vi "Read Test Configuration (INI) File.vi"() -> (1 "Filename":string, 2 "Filepath":path, 3 "Experiments":T1={"Exp 1"={"P2_Sweep_Stop_V"=36.0, "P2_Sweep_Step_V"=1.0, "Experiment Name"="", "Resistance Threshold"=1.0, "P1_Fixed_Voltage"=36.0, "P2_Sweep_Start_V"=36.0}, "Exp 3"={"P2_Sweep_Stop_V"=36.0, "P2_Sweep_Step_V"=1.0, "Experiment Name"="", "Resistance Threshold"=1.0, "P1_Fixed_Voltage"=36.0, "P2_Sweep_Start_V"=36.0}, "Exp 2"={"P2_Sweep_Stop_V"=36.0, "P2_Sweep_Step_V"=1.0, "Experiment Name"="", "Resistance Threshold"=1.0, "P1_Fixed_Voltage"=36.0, "P2_Sweep_Start_V"=36.0}, "Exp 4"={"P2_Sweep_Stop_V"=36.0, "P2_Sweep_Step_V"=1.0, "Experiment Name"="", "Resistance Threshold"=1.0, "P1_Fixed_Voltage"=36.0, "P2_Sweep_Start_V"=36.0}})   [LabVIEW 2013]
doc: "Read Test Configuration file. Set Cluster Output which SDR will choose from later."
uses:
  Support/Controls/Multiple Exp Setup.ctl
  Support/Controls/Individual User Inputs.ctl
  <vilib>/Utility/config.llb/Read Key (Double).vi
  <vilib>/Utility/config.llb/Read Key (String).vi
  <vilib>/Utility/config.llb/Read Key (Path).vi
  <vilib>/Utility/config.llb/NI_LVConfig.lvlib
panel:
  # "Test Settings"
  # "Make the Stop and Step Negative \nfor negative sweep"
  # "Calculation Settings"
  # "Test Settings"
  # "Make the Stop and Step Negative \nfor negative sweep"
  # "Calculation Settings"
  # "Test Settings"
  # "Make the Stop and Step Negative \nfor negative sweep"
  # "Calculation Settings"
  # "Test Settings"
  # "Make the Stop and Step Negative \nfor negative sweep"
  # "Calculation Settings"
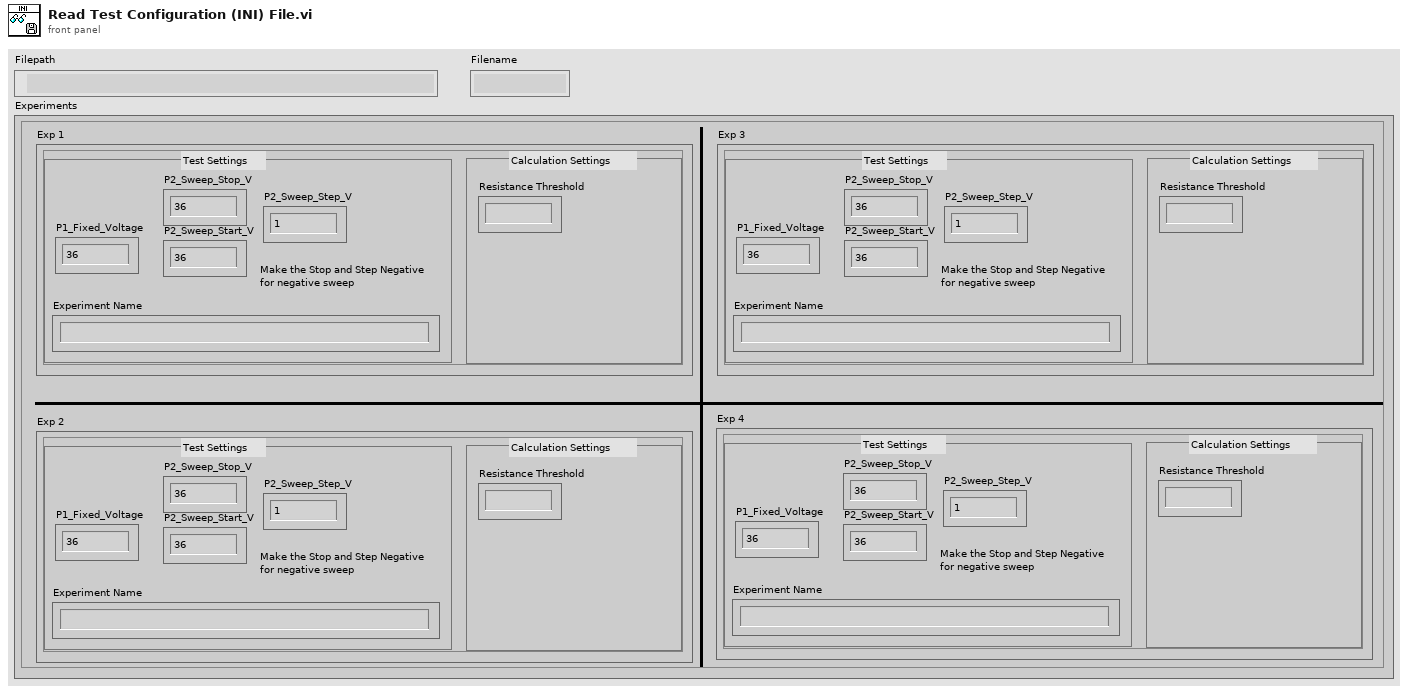
[diagram p1: front panel]
types:
  T1 = typedef "Multiple Exp Setup.ctl" = cluster{"Exp 1":T2, "Exp 3":T2, "Exp 2":T2, "Exp 4":T2}
  T2 = typedef "Individual User Inputs.ctl" = cluster{"P2_Sweep_Stop_V":dbl, "P2_Sweep_Step_V":dbl, "Experiment Name":string, "Resistance Threshold":dbl, "P1_Fixed_Voltage":dbl, "P2_Sweep_Start_V":dbl}
  T3 = typedef "NI_LVConfig.lvlib/Config Data RefNum.ctl" = refnum<k1>
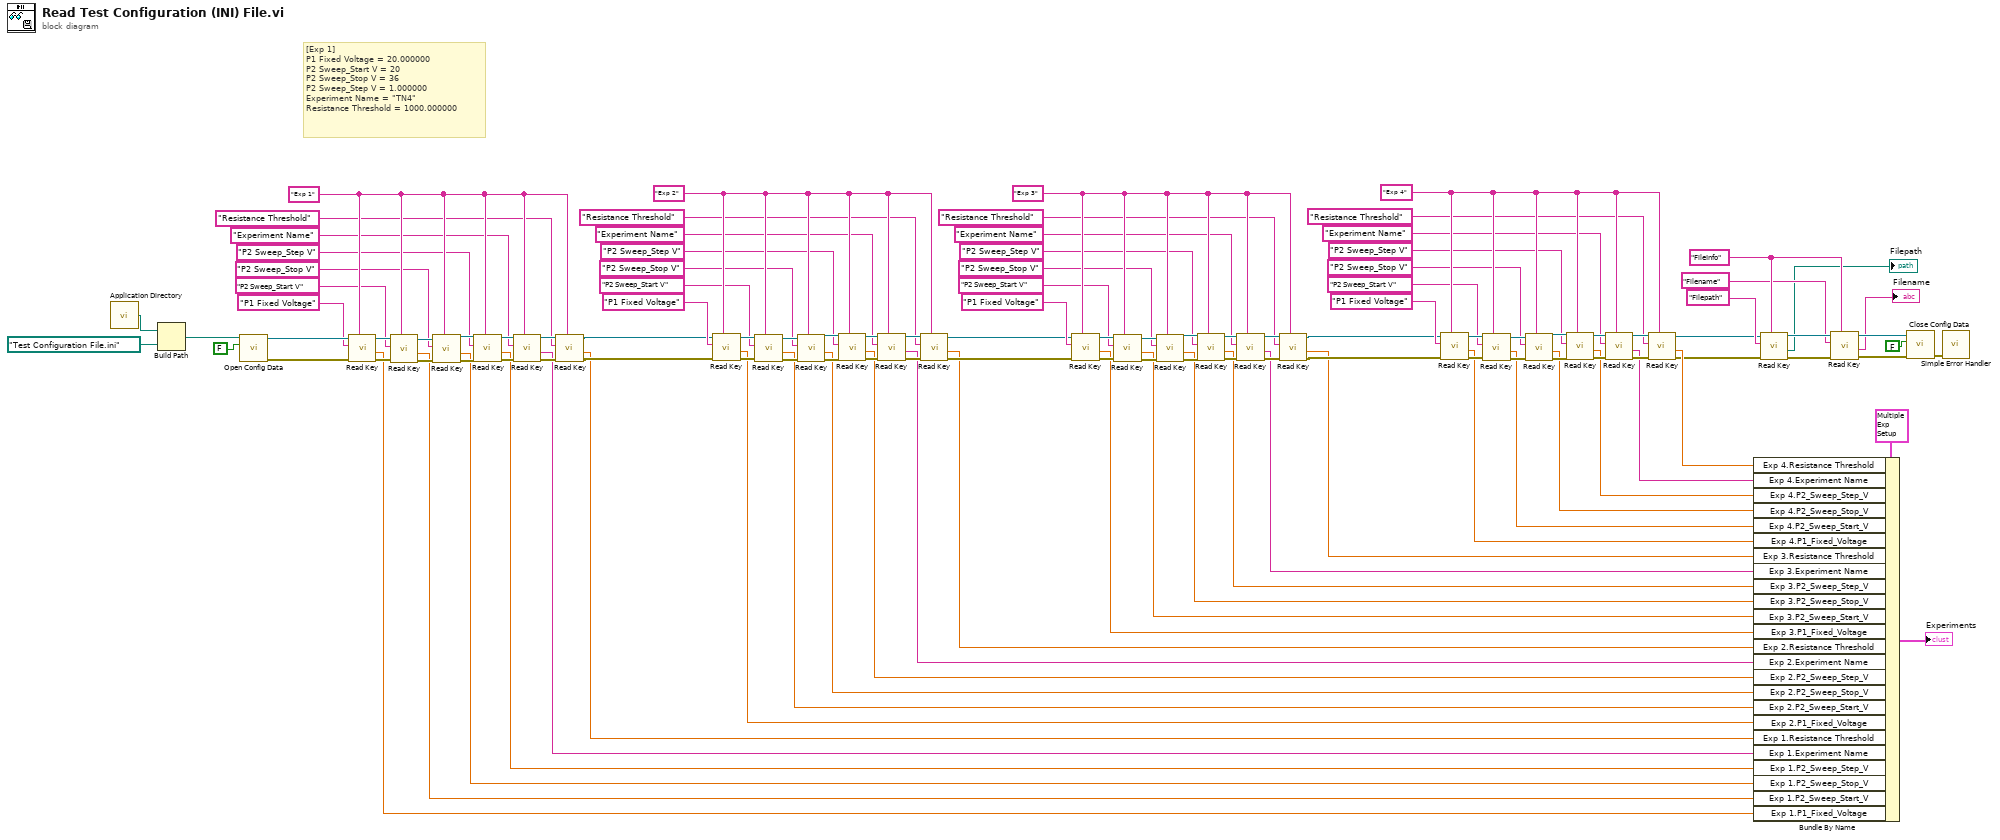
[diagram p0: block diagram]
diagram:
  w8 = "FileInfo" ("section")
  w44 = "Exp 4" ("section")
  w63 = "Exp 3" ("section")
  w82 = "Exp 2" ("section")
  w99 = "Exp 1" ("section")
  # "[Exp 1]\nP1 Fixed Voltage = 20.000000\nP2 Sweep_Start V = 20 \nP2 Sweep_Stop V = 36   \nP2 Sweep_Step V = 1.000000    \nExperiment Name = \"TN4\"\nResistance Threshold = 1000.000000"
  n1 = call <vilib>:"Application Directory.vi"() -> ("Application Directory"=w106:path)
  n2 = Build Path(base path=w106, name or relative path=path "Test Configuration File.ini" ("default name")) -> (appended path=w115:path)
  n3 = call <vilib>:"Open Config Data.vi"("create file if necessary (T)"=FALSE ("create file if necessary? (T)"), "configuration file path"=w115) -> ("error out"=w101:errorcluster, "refnum"=w102:T3)  [unwired: 7 in, 1 out]
  n4 = call-poly <vilib>:"Read Key.vi"("section"=w99, "error in (no error)"=w101, "key"="P1 Fixed Voltage" ("Key 1"), "refnum"=w102) -> ("error out"=w100:errorcluster, "value"=w12:dbl, "refnum out"=w103:T3)  [unwired: 4 in, 1 out]
  n5 = call-poly <vilib>:"Read Key.vi"("section"=w99, "error in (no error)"=w100, "key"="P2 Sweep_Start V" ("Key 2"), "refnum"=w103) -> ("error out"=w105:errorcluster, "value"=w13:dbl, "refnum out"=w104:T3)  [unwired: 4 in, 1 out]
  n6 = call-poly <vilib>:"Read Key.vi"("section"=w99, "error in (no error)"=w105, "key"="P2 Sweep_Stop V" ("Key 2"), "refnum"=w104) -> ("error out"=w112:errorcluster, "value"=w14:dbl, "refnum out"=w111:T3)  [unwired: 4 in, 1 out]
  n7 = call-poly <vilib>:"Read Key.vi"("section"=w99, "error in (no error)"=w112, "key"="P2 Sweep_Step V" ("Key 2"), "refnum"=w111) -> ("error out"=w113:errorcluster, "value"=w15:dbl, "refnum out"=w114:T3)  [unwired: 1 in, 4 out]
  n8 = call-poly <vilib>:"Read Key.vi"("section"=w99, "error in (no error)"=w113, "key"="Experiment Name" ("Key 3"), "refnum"=w114) -> ("error out"=w109:errorcluster, "value"=w16:string, "refnum out"=w108:T3)  [unwired: 2 in, 3 out]
  n9 = call-poly <vilib>:"Read Key.vi"("section"=w99, "error in (no error)"=w109, "key"="Resistance Threshold" ("Key 3"), "refnum"=w108) -> ("error out"=w75:errorcluster, "value"=w17:dbl, "refnum out"=w74:T3)  [unwired: 1 in, 4 out]
  n10 = call-poly <vilib>:"Read Key.vi"("section"=w82, "error in (no error)"=w75, "key"="P1 Fixed Voltage" ("Key 1"), "refnum"=w74) -> ("error out"=w83:errorcluster, "value"=w18:dbl, "refnum out"=w84:T3)  [unwired: 4 in, 1 out]
  n11 = call-poly <vilib>:"Read Key.vi"("section"=w82, "error in (no error)"=w83, "key"="P2 Sweep_Start V" ("Key 2"), "refnum"=w84) -> ("error out"=w86:errorcluster, "value"=w19:dbl, "refnum out"=w85:T3)  [unwired: 4 in, 1 out]
  n12 = call-poly <vilib>:"Read Key.vi"("section"=w82, "error in (no error)"=w86, "key"="P2 Sweep_Stop V" ("Key 2"), "refnum"=w85) -> ("error out"=w90:errorcluster, "value"=w20:dbl, "refnum out"=w89:T3)  [unwired: 4 in, 1 out]
  n13 = call-poly <vilib>:"Read Key.vi"("section"=w82, "error in (no error)"=w90, "key"="P2 Sweep_Step V" ("Key 2"), "refnum"=w89) -> ("error out"=w91:errorcluster, "value"=w21:dbl, "refnum out"=w92:T3)  [unwired: 1 in, 4 out]
  n14 = call-poly <vilib>:"Read Key.vi"("section"=w82, "error in (no error)"=w91, "key"="Experiment Name" ("Key 3"), "refnum"=w92) -> ("error out"=w88:errorcluster, "value"=w22:string, "refnum out"=w87:T3)  [unwired: 2 in, 3 out]
  n15 = call-poly <vilib>:"Read Key.vi"("section"=w82, "error in (no error)"=w88, "key"="Resistance Threshold" ("Key 3"), "refnum"=w87) -> ("error out"=w56:errorcluster, "value"=w23:dbl, "refnum out"=w55:T3)  [unwired: 1 in, 4 out]
  n16 = call-poly <vilib>:"Read Key.vi"("section"=w63, "error in (no error)"=w56, "key"="P1 Fixed Voltage" ("Key 1"), "refnum"=w55) -> ("error out"=w64:errorcluster, "value"=w24:dbl, "refnum out"=w65:T3)  [unwired: 4 in, 1 out]
  n17 = call-poly <vilib>:"Read Key.vi"("section"=w63, "error in (no error)"=w64, "key"="P2 Sweep_Start V" ("Key 2"), "refnum"=w65) -> ("error out"=w67:errorcluster, "value"=w25:dbl, "refnum out"=w66:T3)  [unwired: 4 in, 1 out]
  n18 = call-poly <vilib>:"Read Key.vi"("section"=w63, "error in (no error)"=w67, "key"="P2 Sweep_Stop V" ("Key 2"), "refnum"=w66) -> ("error out"=w71:errorcluster, "value"=w26:dbl, "refnum out"=w70:T3)  [unwired: 4 in, 1 out]
  n19 = call-poly <vilib>:"Read Key.vi"("section"=w63, "error in (no error)"=w71, "key"="P2 Sweep_Step V" ("Key 2"), "refnum"=w70) -> ("error out"=w72:errorcluster, "value"=w27:dbl, "refnum out"=w73:T3)  [unwired: 1 in, 4 out]
  n20 = call-poly <vilib>:"Read Key.vi"("section"=w63, "error in (no error)"=w72, "key"="Experiment Name" ("Key 3"), "refnum"=w73) -> ("error out"=w69:errorcluster, "value"=w28:string, "refnum out"=w68:T3)  [unwired: 2 in, 3 out]
  n21 = call-poly <vilib>:"Read Key.vi"("section"=w63, "error in (no error)"=w69, "key"="Resistance Threshold" ("Key 3"), "refnum"=w68) -> ("error out"=w37:errorcluster, "value"=w29:dbl, "refnum out"=w36:T3)  [unwired: 1 in, 4 out]
  n22 = call-poly <vilib>:"Read Key.vi"("section"=w44, "error in (no error)"=w37, "key"="P1 Fixed Voltage" ("Key 1"), "refnum"=w36) -> ("error out"=w45:errorcluster, "value"=w30:dbl, "refnum out"=w46:T3)  [unwired: 4 in, 1 out]
  n23 = call-poly <vilib>:"Read Key.vi"("section"=w44, "error in (no error)"=w45, "key"="P2 Sweep_Start V" ("Key 2"), "refnum"=w46) -> ("error out"=w48:errorcluster, "value"=w31:dbl, "refnum out"=w47:T3)  [unwired: 4 in, 1 out]
  n24 = call-poly <vilib>:"Read Key.vi"("section"=w44, "error in (no error)"=w48, "key"="P2 Sweep_Stop V" ("Key 2"), "refnum"=w47) -> ("error out"=w52:errorcluster, "value"=w32:dbl, "refnum out"=w51:T3)  [unwired: 4 in, 1 out]
  n25 = call-poly <vilib>:"Read Key.vi"("section"=w44, "error in (no error)"=w52, "key"="P2 Sweep_Step V" ("Key 2"), "refnum"=w51) -> ("error out"=w53:errorcluster, "value"=w33:dbl, "refnum out"=w54:T3)  [unwired: 1 in, 4 out]
  n26 = call-poly <vilib>:"Read Key.vi"("section"=w44, "error in (no error)"=w53, "key"="Experiment Name" ("Key 3"), "refnum"=w54) -> ("error out"=w50:errorcluster, "value"=w34:string, "refnum out"=w49:T3)  [unwired: 2 in, 3 out]
  n27 = call-poly <vilib>:"Read Key.vi"("section"=w44, "error in (no error)"=w50, "key"="Resistance Threshold" ("Key 3"), "refnum"=w49) -> ("error out"=w6:errorcluster, "value"=w35:dbl, "refnum out"=w5:T3)  [unwired: 1 in, 4 out]
  n28 = Bundle By Name(cluster=T1 {"Exp 1"={"P2_Sweep_Stop_V"=36.0, "P2_Sweep_Step_V"=1.0, "Experiment Name"="", "Resistance Threshold"=1.0, "P1_Fixed_Voltage"=0.0, "P2_Sweep_Start_V"=0.0}, "Exp 3"={"P2_Sweep_Stop_V"=36.0, "P2_Sweep_Step_V"=1.0, "Experiment Name"="", "Resistance Threshold"=1.0, "P1_Fixed_Voltage"=0.0, "P2_Sweep_Start_V"=0.0}, "Exp 2"={"P2_Sweep_Stop_V"=36.0, "P2_Sweep_Step_V"=1.0, "Experiment Name"="", "Resistance Threshold"=1.0, "P1_Fixed_Voltage"=0.0, "P2_Sweep_Start_V"=0.0}, "Exp 4"={"P2_Sweep_Stop_V"=36.0, "P2_Sweep_Step_V"=1.0, "Experiment Name"="", "Resistance Threshold"=1.0, "P1_Fixed_Voltage"=0.0, "P2_Sweep_Start_V"=0.0}} ("Experiments"), "Exp 4.Resistance Threshold"=w35, "Exp 4.Experiment Name"=w34, "Exp 4.P2_Sweep_Step_V"=w33, "Exp 4.P2_Sweep_Stop_V"=w32, "Exp 4.P2_Sweep_Start_V"=w31, "Exp 4.P1_Fixed_Voltage"=w30, "Exp 3.Resistance Threshold"=w29, "Exp 3.Experiment Name"=w28, "Exp 3.P2_Sweep_Step_V"=w27, "Exp 3.P2_Sweep_Stop_V"=w26, "Exp 3.P2_Sweep_Start_V"=w25, "Exp 3.P1_Fixed_Voltage"=w24, "Exp 2.Resistance Threshold"=w23, "Exp 2.Experiment Name"=w22, "Exp 2.P2_Sweep_Step_V"=w21, "Exp 2.P2_Sweep_Stop_V"=w20, "Exp 2.P2_Sweep_Start_V"=w19, "Exp 2.P1_Fixed_Voltage"=w18, "Exp 1.Resistance Threshold"=w17, "Exp 1.Experiment Name"=w16, "Exp 1.P2_Sweep_Step_V"=w15, "Exp 1.P2_Sweep_Stop_V"=w14, "Exp 1.P2_Sweep_Start_V"=w13, "Exp 1.P1_Fixed_Voltage"=w12) -> (→"Experiments":T1)
  n29 = call-poly <vilib>:"Read Key.vi"("section"=w8, "error in (no error)"=w6, "key"="Filepath" ("Key 1"), "refnum"=w5) -> ("error out"=w9:errorcluster, "value"=→"Filepath":path, "refnum out"=w10:T3)  [unwired: 4 in, 1 out]
  n30 = call-poly <vilib>:"Read Key.vi"("section"=w8, "error in (no error)"=w9, "key"="Filename" ("Key 1"), "refnum"=w10) -> ("error out"=w3:errorcluster, "value"=→"Filename":string, "refnum out"=w4:T3)  [unwired: 4 in, 1 out]
  n31 = call <vilib>:"Close Config Data.vi"("error in (no error)"=w3, "write file if changed (T)"=FALSE ("write configuration file? (T)"), "refnum"=w4) -> ("error out"=w117:errorcluster)  [unwired: 8 out]
  n32 = call <vilib>:"Simple Error Handler.vi"("error in (no error)"=w117) -> ()  [unwired: 1 in, 8 out]
